vi "Measure vs B2Dv7.vi"() -> ()   [LabVIEW 2009]
doc: "This VI is an example operator panel.\n\nThe VI contains a table for the field values that may be configured manually, or loaded by checking the \"Prompt for File\" box. The data file should contain 3 columns of data, with each column delimited by a tab character.\n\nBefore the VI is executed, set the desired field units and coordinate system. Once the VI is started, follow the directions in the STATUS indicator to operate. Once a field value is achieved, it will be held indefinitely with no user intervention.\n\nThe present field is displayed in the selected units and coordinate system. The present field is queried once per second.\n\nIf a field point is specified that is outside the limits for the magnet, the VI will abort execution."
uses:
  <vilib>/Utility/file.llb/Read From Spreadsheet File (DBL).vi
panel:
  out "appended array":dbl[](array[numeric])=[0.2032200002460388, 90.00281939668669, 0.0, 0.0, 0.0, 0.0, 0.0, 0.0, 0.0, 0.0, -5.519596, 3403272764.31614]
  in  "Nr. of Accumulations":i32=5
  in  "X Axis":enum16{"B", "phi"}(ring)
  in  "Y Axis":T1(ring)=enum."HP (V)"
  out "XY Graph":T2(graph)={"measured data"=[0.10347000048323185, 0.19641000025456953, 0.29707, 0.396860000125989, 0.49694000010061584, 0.5974600000836876, 0.69603, 0.7960300000628118, 0.8974500000557136, 0.9966200002006783, 1.0970900000000001, 1.19673, 1.29725, 1.39698, 1.49648, 1.5970800000313075, 1.6969500000000002, 1.796500000027832, 1.8966700000263619, 1.9970400000000001, 2.0967400000238468, 2.196980000022758, 2.2964100000870924, 2.396280000020866, 2.49752000002002, 2.5961200000000004, 2.6964400000185433, 2.79707, 2.8966900000172613, 2.996840000016684, 3.0965000000000003, 3.1975700000000002, 3.29701, 3.39604, 3.496610000014299, 3.5968600000139013, 3.6964300000000003, 3.79707, 3.896600000012832, 3.99675000001251, 4.09672, 4.197190000011912, 4.29626, 4.3964799999999995, 4.496670000000001, 4.597080000010876, 4.696600000010646, 4.796870000010423, 4.896420000010211, 4.996820000010007, 4.903020000000001, 4.802990000010411, 4.703300000010631, 4.602810000043452, 4.50282, 4.403030000011356, 4.303300000011619, 4.203860000000001, 4.103380000012185, 4.002780000012492, 3.90318, 3.80358, 3.7033500000135007, 3.603490000013876, 3.5029500000142733, 3.40296, 3.3031700000605486, 3.2035800000156076, 3.10286, 3.0031200000665974, 2.90348, 2.8030600000000003, 2.7033300000000002, 2.603300000019207, 2.5035000000000003, 2.403530000020803, 2.3033300000000003, 2.2031300000000003, 2.1029400000237763, 2.003560000024956, 1.9032600000262705, 1.8035800000277225, 1.7029600000293605, 1.6035700000311803, 1.5032900000332605, 1.4031900000356332, 1.3032700000383652, 1.20313, 1.10329, 1.00339, 0.90345, 0.8029400000622712, 0.7036, 0.60275, 0.50339, 0.40294, 0.302990000165022, 0.2032200002460388], "measured data"=[-1.563466, -1.08216, -0.70321, -0.409586, -0.269864, -0.025948, 0.180408, 0.261814, 0.30081199999999997, -0.068092, -0.57451, -1.0081479999999998, -2.017134, -2.885122, -3.9488559999999997, -5.384270000000001, -7.012888, -8.998236, -11.360275999999999, -14.308696, -17.92829, -22.338188000000002, -28.965936000000003, -36.3468, -44.4973, -53.671188, -60.597266, -67.282196, -73.833424, -80.22503, -86.434398, -92.21979400000001, -97.86212, -103.22911199999999, -108.601316, -113.677622, -118.671314, -123.51419200000001, -128.272526, -132.90004199999998, -137.67711400000002, -142.21992799999998, -146.755386, -151.024336, -155.5273, -159.64799399999998, -163.87723999999997, -168.28429, -172.573372, -176.459164, -165.88622399999997, -156.948784, -147.825416, -141.431096, -136.35452, -131.8822, -127.589888, -123.29114200000001, -119.12121399999998, -115.08163, -111.252546, -107.22219799999999, -103.221754, -99.245906, -95.414286, -91.35763800000001, -87.32137, -83.26736600000001, -79.067984, -75.06495600000001, -70.80681200000001, -66.649182, -62.36449400000001, -58.344514000000004, -53.993213999999995, -50.057770000000005, -45.802158000000006, -42.018744, -38.010557999999996, -34.145004, -30.535152, -27.03073, -23.526186000000003, -20.238034, -17.346718, -14.648320000000002, -12.144, -9.910048, -7.987274, -6.390732, -5.077078, -4.234354, -3.7365180000000002, -3.579744, -3.8743040000000004, -4.396356, -5.0064459999999995, -5.519596]}
  in  "GPIB HP 2":string="13"
  in  "Wait between \nVectors":bool=TRUE
  in  "FieldRange":dbl=1.0
  in  "Change\nPID\n(DetermineSIMPID.vi)":bool
  in  "Wait between \nVectors (ms)":u32=4000
  out "measured data":dbl[][](array[numeric])=[[0.10347000048323185, 90.00553742914224, 0.0, 0.0, 0.0, 0.0, 0.0, 0.0, 0.0, 0.0, -1.563466, 3403269629.8467245], [0.19641000025456953, 89.99708284815114, 0.0, 0.0, 0.0, 0.0, 0.0, 0.0, 0.0, 0.0, -1.08216, 3403269661.616901], [0.29707, 90.0, 0.0, 0.0, 0.0, 0.0, 0.0, 0.0, 0.0, 0.0, -0.70321, 3403269694.1531544], [0.396860000125989, 90.00144372775037, 0.0, 0.0, 0.0, 0.0, 0.0, 0.0, 0.0, 0.0, -0.409586, 3403269726.399379], [0.49694000010061584, 89.99884702822263, 0.0, 0.0, 0.0, 0.0, 0.0, 0.0, 0.0, 0.0, -0.269864, 3403269759.355674], [0.5974600000836876, 90.00095898938018, 0.0, 0.0, 0.0, 0.0, 0.0, 0.0, 0.0, 0.0, -0.025948, 3403269791.685907], [0.69603, 90.0, 0.0, 0.0, 0.0, 0.0, 0.0, 0.0, 0.0, 0.0, 0.180408, 3403269823.3570733], [0.7960300000628118, 89.99928023090197, 0.0, 0.0, 0.0, 0.0, 0.0, 0.0, 0.0, 0.0, 0.261814, 3403269855.5922966], [0.8974500000557136, 90.00063842865353, 0.0, 0.0, 0.0, 0.0, 0.0, 0.0, 0.0, 0.0, 0.30081199999999997, 3403269888.02954], [0.9966200002006783, 90.0011498019206, 0.0, 0.0, 0.0, 0.0, 0.0, 0.0, 0.0, 0.0, -0.068092, 3403269919.970734], [1.0970900000000001, 90.0, 0.0, 0.0, 0.0, 0.0, 0.0, 0.0, 0.0, 0.0, -0.57451, 3403269952.1809545], [1.19673, 90.0, 0.0, 0.0, 0.0, 0.0, 0.0, 0.0, 0.0, 0.0, -1.0081479999999998, 3403269983.93713], [1.29725, 90.0, 0.0, 0.0, 0.0, 0.0, 0.0, 0.0, 0.0, 0.0, -2.017134, 3403270016.8654222], [1.39698, 90.0, 0.0, 0.0, 0.0, 0.0, 0.0, 0.0, 0.0, 0.0, -2.885122, 3403270049.372673], [1.49648, 90.0, 0.0, 0.0, 0.0, 0.0, 0.0, 0.0, 0.0, 0.0, -3.9488559999999997, 3403270081.84692], [1.5970800000313075, 89.9996412466532, 0.0, 0.0, 0.0, 0.0, 0.0, 0.0, 0.0, 0.0, -5.384270000000001, 3403270114.493184], [1.6969500000000002, 90.0, 0.0, 0.0, 0.0, 0.0, 0.0, 0.0, 0.0, 0.0, -7.012888, 3403270146.7094054], [1.796500000027832, 89.9996810699721, 0.0, 0.0, 0.0, 0.0, 0.0, 0.0, 0.0, 0.0, -8.998236, 3403270178.7226067], [1.8966700000263619, 90.00030208618006, 0.0, 0.0, 0.0, 0.0, 0.0, 0.0, 0.0, 0.0, -11.360275999999999, 3403270210.912825], [1.9970400000000001, 90.0, 0.0, 0.0, 0.0, 0.0, 0.0, 0.0, 0.0, 0.0, -14.308696, 3403270243.424076], [2.0967400000238468, 90.00027326125087, 0.0, 0.0, 0.0, 0.0, 0.0, 0.0, 0.0, 0.0, -17.92829, 3403270275.8403172], [2.196980000022758, 89.99973920664041, 0.0, 0.0, 0.0, 0.0, 0.0, 0.0, 0.0, 0.0, -22.338188000000002, 3403270308.229556], [2.2964100000870924, 89.99950099695167, 0.0, 0.0, 0.0, 0.0, 0.0, 0.0, 0.0, 0.0, -28.965936000000003, 3403270340.8998227], [2.396280000020866, 90.00023910302433, 0.0, 0.0, 0.0, 0.0, 0.0, 0.0, 0.0, 0.0, -36.3468, 3403270373.3240647], [2.49752000002002, 90.00022941069346, 0.0, 0.0, 0.0, 0.0, 0.0, 0.0, 0.0, 0.0, -44.4973, 3403270405.667299], [2.5961200000000004, 90.0, 0.0, 0.0, 0.0, 0.0, 0.0, 0.0, 0.0, 0.0, -53.671188, 3403270437.5914907], [2.6964400000185433, 90.00021248675851, 0.0, 0.0, 0.0, 0.0, 0.0, 0.0, 0.0, 0.0, -60.597266, 3403270469.938725], [2.79707, 90.0, 0.0, 0.0, 0.0, 0.0, 0.0, 0.0, 0.0, 0.0, -67.282196, 3403270502.9180226], [2.8966900000172613, 89.99980220258463, 0.0, 0.0, 0.0, 0.0, 0.0, 0.0, 0.0, 0.0, -73.833424, 3403270534.6661973], [2.996840000016684, 90.00019118731568, 0.0, 0.0, 0.0, 0.0, 0.0, 0.0, 0.0, 0.0, -80.22503, 3403270567.0204325], [3.0965000000000003, 90.0, 0.0, 0.0, 0.0, 0.0, 0.0, 0.0, 0.0, 0.0, -86.434398, 3403270599.029633], [3.1975700000000002, 90.0, 0.0, 0.0, 0.0, 0.0, 0.0, 0.0, 0.0, 0.0, -92.21979400000001, 3403270631.613891], [3.29701, 90.0, 0.0, 0.0, 0.0, 0.0, 0.0, 0.0, 0.0, 0.0, -97.86212, 3403270663.7301025], [3.39604, 90.0, 0.0, 0.0, 0.0, 0.0, 0.0, 0.0, 0.0, 0.0, -103.22911199999999, 3403270695.7623053], [3.496610000014299, 89.9998361390618, 0.0, 0.0, 0.0, 0.0, 0.0, 0.0, 0.0, 0.0, -108.601316, 3403270727.8155103], [3.5968600000139013, 89.99984070611725, 0.0, 0.0, 0.0, 0.0, 0.0, 0.0, 0.0, 0.0, -113.677622, 3403270760.053734], [3.6964300000000003, 90.0, 0.0, 0.0, 0.0, 0.0, 0.0, 0.0, 0.0, 0.0, -118.671314, 3403270792.41597], [3.79707, 90.0, 0.0, 0.0, 0.0, 0.0, 0.0, 0.0, 0.0, 0.0, -123.51419200000001, 3403270824.9382215], [3.896600000012832, 89.99985295955574, 0.0, 0.0, 0.0, 0.0, 0.0, 0.0, 0.0, 0.0, -128.272526, 3403270857.4414716], [3.99675000001251, 90.00014335592547, 0.0, 0.0, 0.0, 0.0, 0.0, 0.0, 0.0, 0.0, -132.90004199999998, 3403270889.768704], [4.09672, 90.0, 0.0, 0.0, 0.0, 0.0, 0.0, 0.0, 0.0, 0.0, -137.67711400000002, 3403270922.309958], [4.197190000011912, 89.99986349014576, 0.0, 0.0, 0.0, 0.0, 0.0, 0.0, 0.0, 0.0, -142.21992799999998, 3403270954.8822145], [4.29626, 90.0, 0.0, 0.0, 0.0, 0.0, 0.0, 0.0, 0.0, 0.0, -146.755386, 3403270987.409467], [4.3964799999999995, 90.0, 0.0, 0.0, 0.0, 0.0, 0.0, 0.0, 0.0, 0.0, -151.024336, 3403271020.102736], [4.496670000000001, 90.0, 0.0, 0.0, 0.0, 0.0, 0.0, 0.0, 0.0, 0.0, -155.5273, 3403271052.174943], [4.597080000010876, 90.00012463515866, 0.0, 0.0, 0.0, 0.0, 0.0, 0.0, 0.0, 0.0, -159.64799399999998, 3403271084.9372187], [4.696600000010646, 89.99987800583504, 0.0, 0.0, 0.0, 0.0, 0.0, 0.0, 0.0, 0.0, -163.87723999999997, 3403271116.9074154], [4.796870000010423, 89.99988055590518, 0.0, 0.0, 0.0, 0.0, 0.0, 0.0, 0.0, 0.0, -168.28429, 3403271149.044629], [4.896420000010211, 89.99988298434465, 0.0, 0.0, 0.0, 0.0, 0.0, 0.0, 0.0, 0.0, -172.573372, 3403271180.869811], [4.996820000010007, 90.00011466448564, 0.0, 0.0, 0.0, 0.0, 0.0, 0.0, 0.0, 0.0, -176.459164, 3403271213.3300567], [4.903020000000001, 90.0, 0.0, 0.0, 0.0, 0.0, 0.0, 0.0, 0.0, 0.0, -165.88622399999997, 3403271245.606284], [4.802990000010411, 90.00011929189841, 0.0, 0.0, 0.0, 0.0, 0.0, 0.0, 0.0, 0.0, -156.948784, 3403271277.7614994], [4.703300000010631, 90.0001218203804, 0.0, 0.0, 0.0, 0.0, 0.0, 0.0, 0.0, 0.0, -147.825416, 3403271310.397763], [4.602810000043452, 90.00024896000275, 0.0, 0.0, 0.0, 0.0, 0.0, 0.0, 0.0, 0.0, -141.431096, 3403271342.6319857], [4.50282, 90.0, 0.0, 0.0, 0.0, 0.0, 0.0, 0.0, 0.0, 0.0, -136.35452, 3403271374.9822206], [4.403030000011356, 89.99986987193022, 0.0, 0.0, 0.0, 0.0, 0.0, 0.0, 0.0, 0.0, -131.8822, 3403271407.48147], [4.303300000011619, 89.99986685618128, 0.0, 0.0, 0.0, 0.0, 0.0, 0.0, 0.0, 0.0, -127.589888, 3403271439.4496665], [4.203860000000001, 90.0, 0.0, 0.0, 0.0, 0.0, 0.0, 0.0, 0.0, 0.0, -123.29114200000001, 3403271471.840905], [4.103380000012185, 89.9998603693065, 0.0, 0.0, 0.0, 0.0, 0.0, 0.0, 0.0, 0.0, -119.12121399999998, 3403271503.7760987], [4.002780000012492, 89.9998568600335, 0.0, 0.0, 0.0, 0.0, 0.0, 0.0, 0.0, 0.0, -115.08163, 3403271536.004321], [3.90318, 90.0, 0.0, 0.0, 0.0, 0.0, 0.0, 0.0, 0.0, 0.0, -111.252546, 3403271568.6915894], [3.80358, 90.0, 0.0, 0.0, 0.0, 0.0, 0.0, 0.0, 0.0, 0.0, -107.22219799999999, 3403271600.5907793], [3.7033500000135007, 89.99984528662019, 0.0, 0.0, 0.0, 0.0, 0.0, 0.0, 0.0, 0.0, -103.221754, 3403271633.2210417], [3.603490000013876, 90.00015900080065, 0.0, 0.0, 0.0, 0.0, 0.0, 0.0, 0.0, 0.0, -99.245906, 3403271665.3602552], [3.5029500000142733, 90.00016356436579, 0.0, 0.0, 0.0, 0.0, 0.0, 0.0, 0.0, 0.0, -95.414286, 3403271697.578477], [3.40296, 90.0, 0.0, 0.0, 0.0, 0.0, 0.0, 0.0, 0.0, 0.0, -91.35763800000001, 3403271730.0967283], [3.3031700000605486, 89.99965308609904, 0.0, 0.0, 0.0, 0.0, 0.0, 0.0, 0.0, 0.0, -87.32137, 3403271762.6699853], [3.2035800000156076, 90.0001788492234, 0.0, 0.0, 0.0, 0.0, 0.0, 0.0, 0.0, 0.0, -83.26736600000001, 3403271795.0122194], [3.10286, 90.0, 0.0, 0.0, 0.0, 0.0, 0.0, 0.0, 0.0, 0.0, -79.067984, 3403271827.0044184], [3.0031200000665974, 89.99961842497461, 0.0, 0.0, 0.0, 0.0, 0.0, 0.0, 0.0, 0.0, -75.06495600000001, 3403271859.015619], [2.90348, 90.0, 0.0, 0.0, 0.0, 0.0, 0.0, 0.0, 0.0, 0.0, -70.80681200000001, 3403271891.048822], [2.8030600000000003, 90.0, 0.0, 0.0, 0.0, 0.0, 0.0, 0.0, 0.0, 0.0, -66.649182, 3403271923.7490916], [2.7033300000000002, 90.0, 0.0, 0.0, 0.0, 0.0, 0.0, 0.0, 0.0, 0.0, -62.36449400000001, 3403271956.3823547], [2.603300000019207, 89.99977991096104, 0.0, 0.0, 0.0, 0.0, 0.0, 0.0, 0.0, 0.0, -58.344514000000004, 3403271988.469563], [2.5035000000000003, 90.0, 0.0, 0.0, 0.0, 0.0, 0.0, 0.0, 0.0, 0.0, -53.993213999999995, 3403272020.721788], [2.403530000020803, 90.00023838179474, 0.0, 0.0, 0.0, 0.0, 0.0, 0.0, 0.0, 0.0, -50.057770000000005, 3403272052.866002], [2.3033300000000003, 90.0, 0.0, 0.0, 0.0, 0.0, 0.0, 0.0, 0.0, 0.0, -45.802158000000006, 3403272085.619277], [2.2031300000000003, 90.0, 0.0, 0.0, 0.0, 0.0, 0.0, 0.0, 0.0, 0.0, -42.018744, 3403272118.202535], [2.1029400000237763, 90.00027245560746, 0.0, 0.0, 0.0, 0.0, 0.0, 0.0, 0.0, 0.0, -38.010557999999996, 3403272150.6097755], [2.003560000024956, 90.0002859698712, 0.0, 0.0, 0.0, 0.0, 0.0, 0.0, 0.0, 0.0, -34.145004, 3403272183.1900334], [1.9032600000262705, 89.99969895978735, 0.0, 0.0, 0.0, 0.0, 0.0, 0.0, 0.0, 0.0, -30.535152, 3403272215.6872826], [1.8035800000277225, 90.00031767805983, 0.0, 0.0, 0.0, 0.0, 0.0, 0.0, 0.0, 0.0, -27.03073, 3403272247.8164954], [1.7029600000293605, 89.99966355181853, 0.0, 0.0, 0.0, 0.0, 0.0, 0.0, 0.0, 0.0, -23.526186000000003, 3403272279.875701], [1.6035700000311803, 90.00035730139322, 0.0, 0.0, 0.0, 0.0, 0.0, 0.0, 0.0, 0.0, -20.238034, 3403272312.562969], [1.5032900000332605, 90.00038113590533, 0.0, 0.0, 0.0, 0.0, 0.0, 0.0, 0.0, 0.0, -17.346718, 3403272344.8691993], [1.4031900000356332, 89.99959167483013, 0.0, 0.0, 0.0, 0.0, 0.0, 0.0, 0.0, 0.0, -14.648320000000002, 3403272377.095422], [1.3032700000383652, 90.00043963092462, 0.0, 0.0, 0.0, 0.0, 0.0, 0.0, 0.0, 0.0, -12.144, 3403272409.408653], [1.20313, 90.0, 0.0, 0.0, 0.0, 0.0, 0.0, 0.0, 0.0, 0.0, -9.910048, 3403272441.6508765], [1.10329, 90.0, 0.0, 0.0, 0.0, 0.0, 0.0, 0.0, 0.0, 0.0, -7.987274, 3403272473.618073], [1.00339, 90.0, 0.0, 0.0, 0.0, 0.0, 0.0, 0.0, 0.0, 0.0, -6.390732, 3403272506.1273236], [0.90345, 90.0, 0.0, 0.0, 0.0, 0.0, 0.0, 0.0, 0.0, 0.0, -5.077078, 3403272538.3895497], [0.8029400000622712, 89.99928642514372, 0.0, 0.0, 0.0, 0.0, 0.0, 0.0, 0.0, 0.0, -4.234354, 3403272570.79679], [0.7036, 90.0, 0.0, 0.0, 0.0, 0.0, 0.0, 0.0, 0.0, 0.0, -3.7365180000000002, 3403272602.6849785], [0.60275, 90.0, 0.0, 0.0, 0.0, 0.0, 0.0, 0.0, 0.0, 0.0, -3.579744, 3403272634.934203], [0.50339, 90.0, 0.0, 0.0, 0.0, 0.0, 0.0, 0.0, 0.0, 0.0, -3.8743040000000004, 3403272667.4324527], [0.40294, 90.0, 0.0, 0.0, 0.0, 0.0, 0.0, 0.0, 0.0, 0.0, -4.396356, 3403272699.4946585], [0.302990000165022, 89.99810898777213, 0.0, 0.0, 0.0, 0.0, 0.0, 0.0, 0.0, 0.0, -5.0064459999999995, 3403272731.8768964], [0.2032200002460388, 90.00281939668669, 0.0, 0.0, 0.0, 0.0, 0.0, 0.0, 0.0, 0.0, -5.519596, 3403272764.31614]]
  in  "Notes:":string="Datum: 31.10.11, Uhrzeit: 15:35, T0.3K,PID LOOPP 0.2, I  200: , Filter auf 12dB und 30Hz, PID Dämpfung:  P=0.6, D=6.2E-5, Laser 25°, 20mA, AOM 10mA, Sweep 0.15T/min,Winkelsweep 0.4° Winkelschritte, warten bei jedem Feldpunkt (measurevsB2Dv7.vi))4s, vectorsm3.txt,Kryo auf dem Boden, nach dem Ausbau des Systems, großer Abstand zwischen Faser und Cantilever(3V Signalamplitude)" caption="Notizen:"
  out "Messfile Refnum":refnum<file>
  in  "Measurement File":path=path "D:/UserData/Matthias/Messungen/STO_LAOR103/111104/111104_R103_90deg_M3.txt"
  in  "Sample name:":string="R103"
  in  "HP 1":bool=TRUE
  in  "GPIB HP":string="14"
  in  "HP 2":bool
  in  "LI 3":bool
  in  "GPIB L 3":string="8"
  in  "LI 2":bool
  in  "GPIB L 2":string="8"
  in  "LI 1":bool
  in  "GPIB L 1":string="8"
  out "Number of lines":i32=99
  in  "Operation":u16(ring)=1 items=["Stepwise", "Continous"]
  out "Ramp Rate along Vector (T/min)":dbl=0.24999999999999994 format="%.3f"
  out "Current Ramp Rate Z (T/min)":dbl=0.24999999874949982 format="%.3f"
  out "Current Ramp Rate Y (T/min)":dbl=2.500500087514032e-05 format="%.3f"
  in  "User defined Ramp Rate (T/min)":bool=TRUE
  in  "User defined Ramp Rate (T/min)":dbl=0.25 format="%.3f"
  in  "Z-Axis Communications Config":T3={"GPIB address"=22, "GPIB bus"=1, "connection ID"=refnum, "IP"="111.111.111.1", "Active Comm Interface"=0, "Serial Port"="", "Programmer Type"=0} {"Programmer Type" items=["Model 430", "Model 420"]; "Active Comm Interface" items=["TCP/IP (Model 430 Only)", "RS232", "IEEE488"]}
  in  "Max Ramp Rate - Y Axis (A/s)":dbl=0.055 format="%.3f"
  in  "Max Ramp Rate - Z Axis (A/s)":dbl=0.19 format="%.3f"
  in  "Magnitude Limit (kG)":dbl=45.1 format="%.3f"
  in  "Y-Axis Communications Config":T3={"GPIB address"=22, "GPIB bus"=1, "connection ID"=refnum, "IP"="111.111.111.2", "Active Comm Interface"=0, "Serial Port"="", "Programmer Type"=0} {"Programmer Type" items=["Model 430", "Model 420"]; "Active Comm Interface" items=["TCP/IP (Model 430 Only)", "RS232", "IEEE488"]}
  out "Cartesian Display (T)":T4={"Y-Axis Field (T)"=0.01746, "Z-Axis Field (T)"=0.99986} {"Z-Axis Field (T)" format="%.3f"; "Y-Axis Field (T)" format="%.3f"}
  in  "Starting index":i32=99
  in  "Normal color":u32(colorbox)=11711154
  in  "Highlight color":u32(colorbox)=16711680
  in  "Prompt for File?":bool=TRUE
  out "Continue Execution?":bool=TRUE
  out "error out":T5
  in  "error in":T5
  out "STATUS":string="Zeroing vector."
  in  "Ramping Control":u16(ring)=4 items=["NEXT VECTOR", "RAMPING", "HOLDING", "PAUSE", "ZERO"]
  out "Cartesian Display (kG)":T6 {"Z-Axis Field (kG)" format="%.3f"; "Y-Axis Field (kG)" format="%.3f"}
  in  "Field Values":string[][](table)=[["0.1000", "90.0000"], ["0.2000", "90.0000"], ["0.3000", "90.0000"], ["0.4000", "90.0000"], ["0.5000", "90.0000"], ["0.6000", "90.0000"], ["0.7000", "90.0000"], ["0.8000", "90.0000"], ["0.9000", "90.0000"], ["1.0000", "90.0000"], ["1.1000", "90.0000"], ["1.2000", "90.0000"], ["1.3000", "90.0000"], ["1.4000", "90.0000"], ["1.5000", "90.0000"], ["1.6000", "90.0000"], ["1.7000", "90.0000"], ["1.8000", "90.0000"], ["1.9000", "90.0000"], ["2.0000", "90.0000"], ["2.1000", "90.0000"], ["2.2000", "90.0000"], ["2.3000", "90.0000"], ["2.4000", "90.0000"], ["2.5000", "90.0000"], ["2.6000", "90.0000"], ["2.7000", "90.0000"], ["2.8000", "90.0000"], ["2.9000", "90.0000"], ["3.0000", "90.0000"], ["3.1000", "90.0000"], ["3.2000", "90.0000"], ["3.3000", "90.0000"], ["3.4000", "90.0000"], ["3.5000", "90.0000"], ["3.6000", "90.0000"], ["3.7000", "90.0000"], ["3.8000", "90.0000"], ["3.9000", "90.0000"], ["4.0000", "90.0000"], ["4.1000", "90.0000"], ["4.2000", "90.0000"], ["4.3000", "90.0000"], ["4.4000", "90.0000"], ["4.5000", "90.0000"], ["4.6000", "90.0000"], ["4.7000", "90.0000"], ["4.8000", "90.0000"], ["4.9000", "90.0000"], ["5.0000", "90.0000"], ["4.9000", "90.0000"], ["4.8000", "90.0000"], ["4.7000", "90.0000"], ["4.6000", "90.0000"], ["4.5000", "90.0000"], ["4.4000", "90.0000"], ["4.3000", "90.0000"], ["4.2000", "90.0000"], ["4.1000", "90.0000"], ["4.0000", "90.0000"], ["3.9000", "90.0000"], ["3.8000", "90.0000"], ["3.7000", "90.0000"], ["3.6000", "90.0000"], ["3.5000", "90.0000"], ["3.4000", "90.0000"], ["3.3000", "90.0000"], ["3.2000", "90.0000"], ["3.1000", "90.0000"], ["3.0000", "90.0000"], ["2.9000", "90.0000"], ["2.8000", "90.0000"], ["2.7000", "90.0000"], ["2.6000", "90.0000"], ["2.5000", "90.0000"], ["2.4000", "90.0000"], ["2.3000", "90.0000"], ["2.2000", "90.0000"], ["2.1000", "90.0000"], ["2.0000", "90.0000"], ["1.9000", "90.0000"], ["1.8000", "90.0000"], ["1.7000", "90.0000"], ["1.6000", "90.0000"], ["1.5000", "90.0000"], ["1.4000", "90.0000"], ["1.3000", "90.0000"], ["1.2000", "90.0000"], ["1.1000", "90.0000"], ["1.0000", "90.0000"], ["0.9000", "90.0000"], ["0.8000", "90.0000"], ["0.7000", "90.0000"], ["0.6000", "90.0000"], ["0.5000", "90.0000"], ["0.4000", "90.0000"], ["0.3000", "90.0000"], ["0.2000", "90.0000"], ["0.1000", "90.0000"]]
  out "Switch Heaters":bool=TRUE
  out "Polar Display (T)":T7={"q (degrees)"=90.0, "Field Magnitude (T)"=0.00023} {"Field Magnitude (T)" format="%.3f"; "q (degrees)" format="%.3f"}
  out "Polar Display (kG)":T8 {"Field Magnitude (kG)" format="%.3f"; "q (degrees)" format="%.3f"}
  in  "Coordinate System":u16(ring)=1 items=["Cartesian", "Polar"]
  in  "Magnetic Field Units":u16(ring)=1 items=["kG", "Tesla"]
  # "Measurement Display"
  # "Measurement Settings"
  # "Magnet Settings"
  # "Max Ramp Rate z: 1.27 T/min\nMax Ramp Rate y: 0.17 T/min"
  # "Devices"
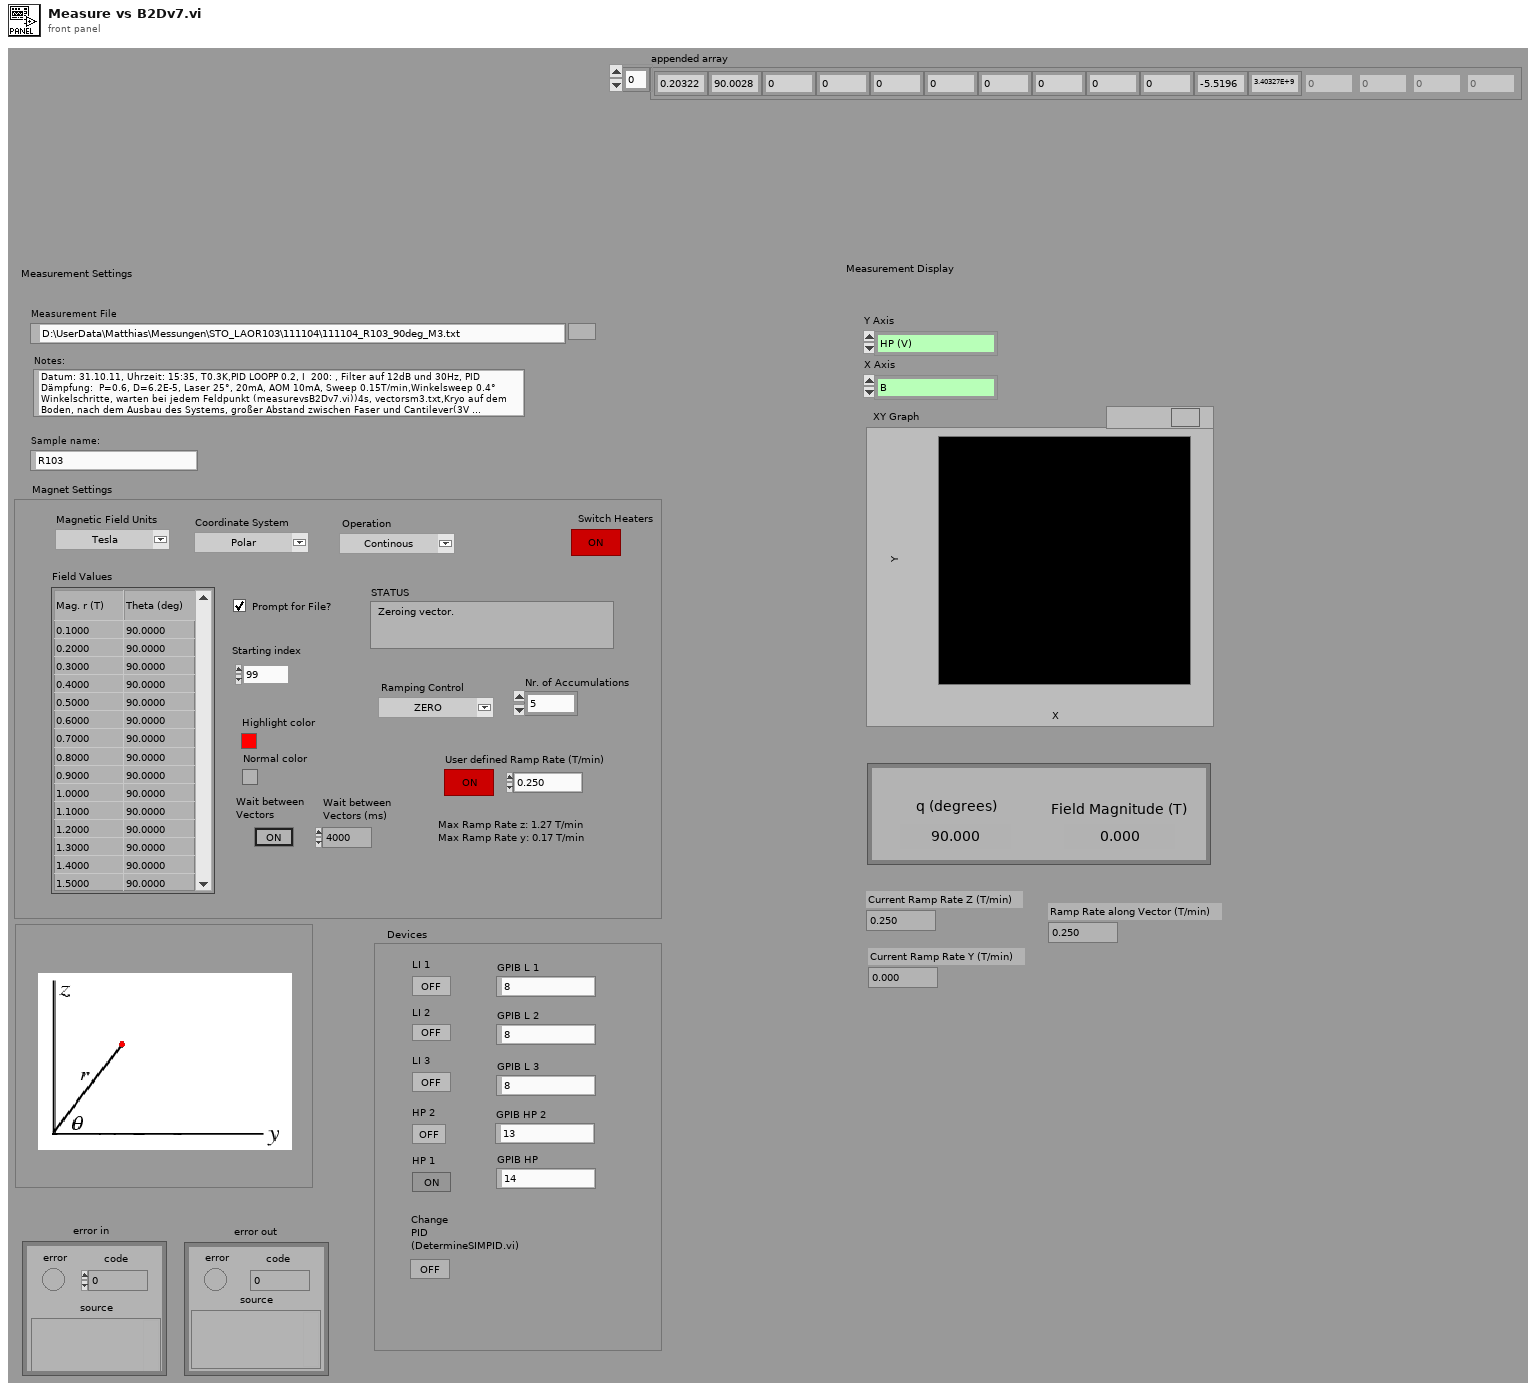
[diagram p1: front panel]
types:
  T1 = enum16{"B", "phi", "LI 1 Vx", "LI 1 phase", "LI 2 Vx", "LI 2 phase", "LI 3 Vx", "LI 3 phase", "LI 4 Vx", "LI 4 phase", "HP (V)"}
  T2 = cluster{"measured data":dbl[], "measured data":dbl[]}
  T3 = cluster{"GPIB address":i16, "GPIB bus":i16, "connection ID":refnum<k5>, "IP":string, "Active Comm Interface":u16, "Serial Port":refnum<visa-resource-name>, "Programmer Type":u16}
  T4 = cluster{"Y-Axis Field (T)":dbl, "Z-Axis Field (T)":dbl}
  T5 = cluster{"error":bool, "code":i32, "source":string}
  T6 = cluster{"Y-Axis Field (kG)":dbl, "Z-Axis Field (kG)":dbl}
  T7 = cluster{"q (degrees)":dbl, "Field Magnitude (T)":dbl}
  T8 = cluster{"q (degrees)":dbl, "Field Magnitude (kG)":dbl}
  T9 = enum16{"", "RAMPING", "HOLDING", "PAUSED", "MANUAL UP", "MANUAL DOWN", "ZEROING CURRENT", "QUENCH DETECTED", "HEATING SWITCH"}
  T10 = enum16{"", "RAMPING", "HOLDING", "PAUSED", "MANUAL UP", "MANUAL DOWN", "ZEROING CURRENT", "QUENCH DETECTED", "HEATING SWITCH", "AT ZER0", "COOLING SWITCH"}
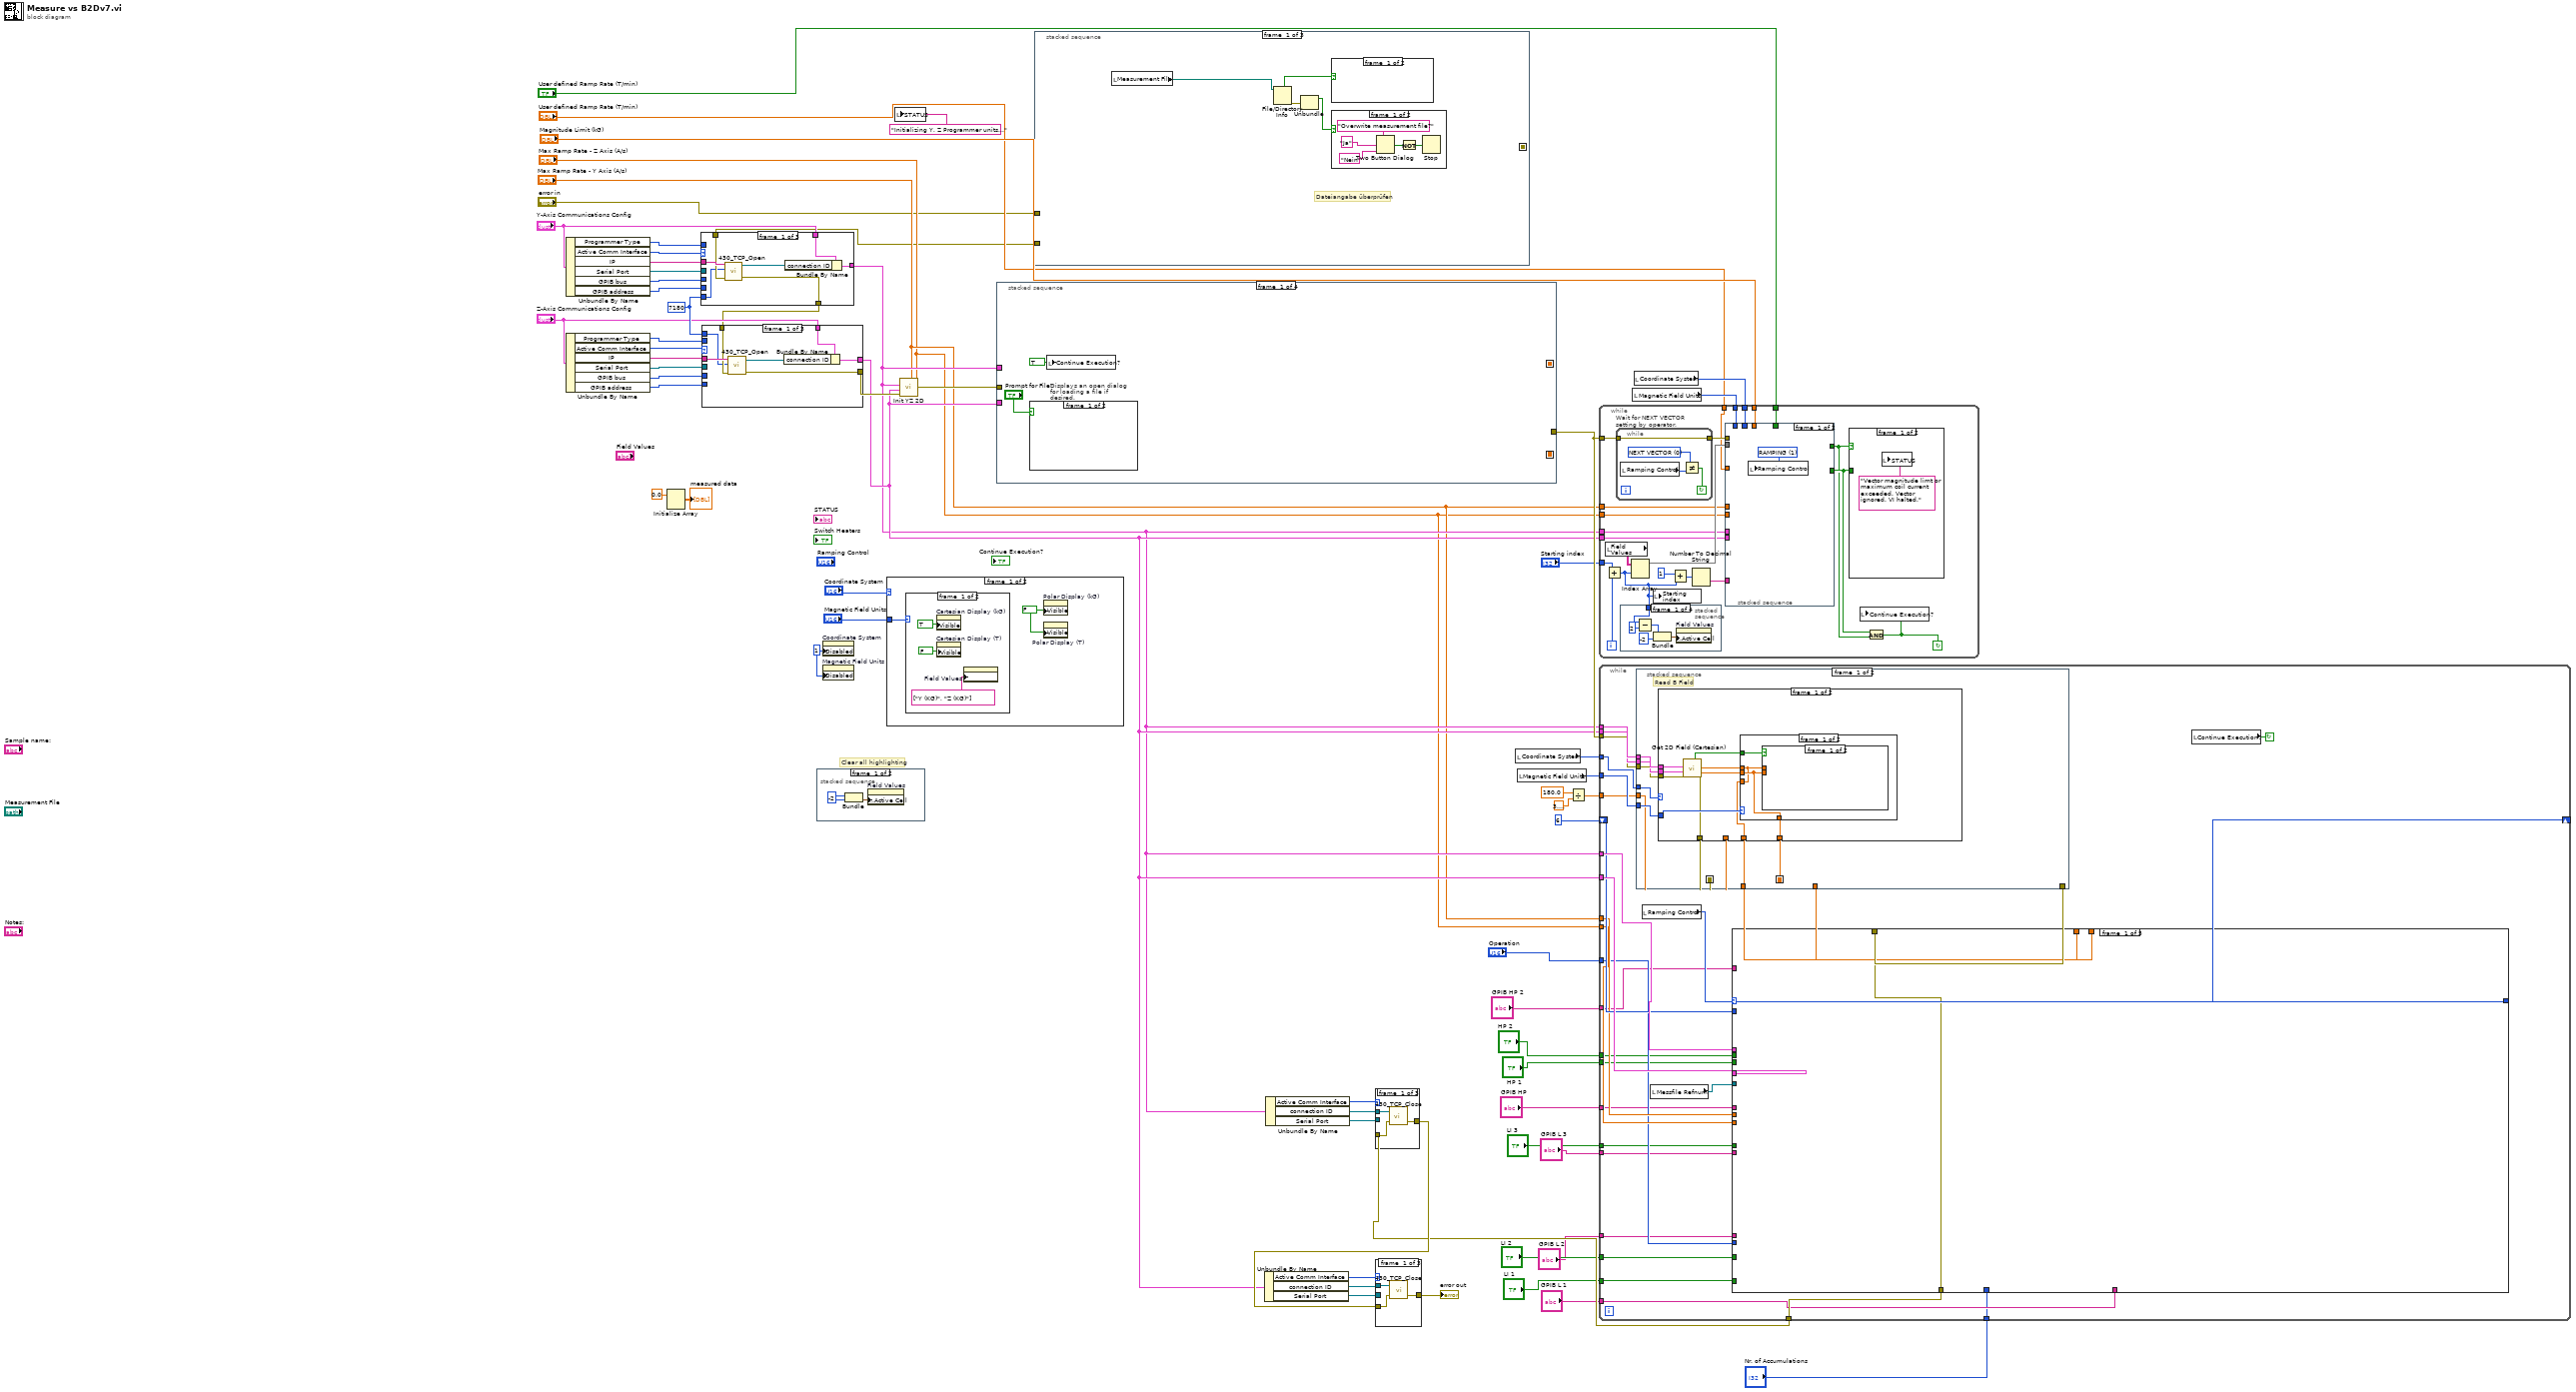
[diagram p0: block diagram]
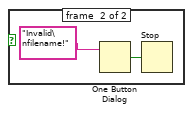
[diagram p3: hidden frame]
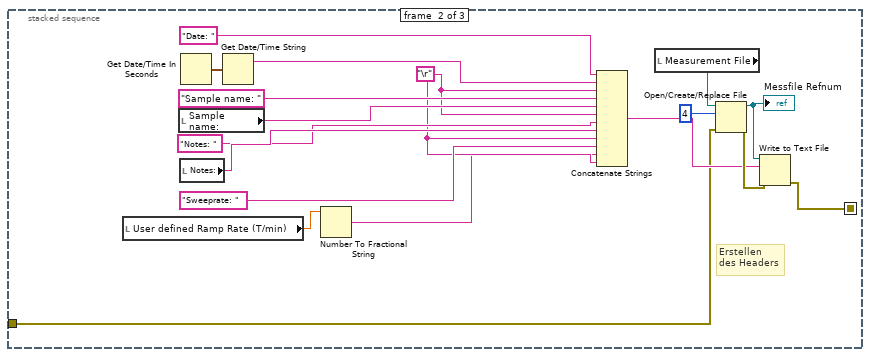
[diagram p4: hidden frame]
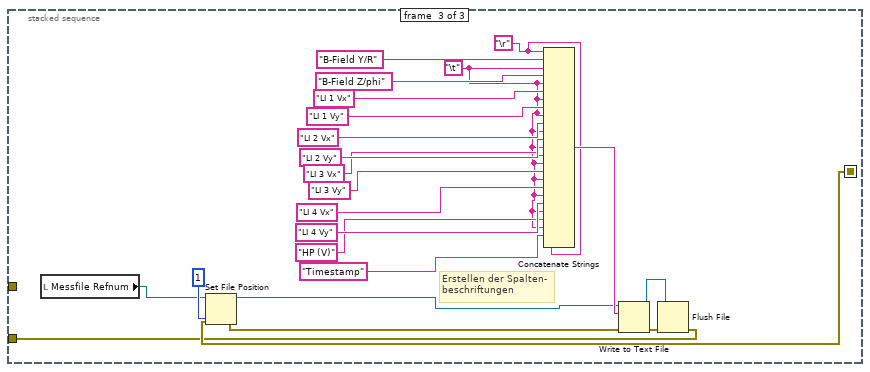
[diagram p5: hidden frame]
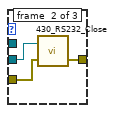
[diagram p6: hidden frame]
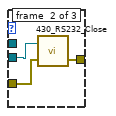
[diagram p8: hidden frame]
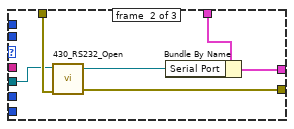
[diagram p10: hidden frame]
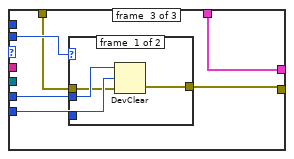
[diagram p11: hidden frame]
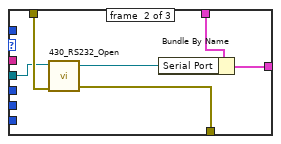
[diagram p13: hidden frame]
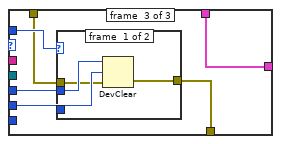
[diagram p14: hidden frame]
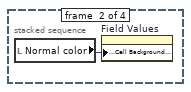
[diagram p16: hidden frame]
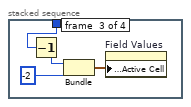
[diagram p17: hidden frame]
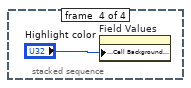
[diagram p18: hidden frame]
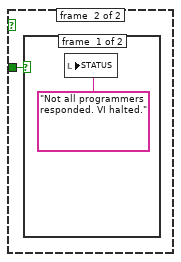
[diagram p19: hidden frame]
diagram:
  w49 = 7180 ("TCP Port")
  w62 = u8 1 ("Write Attribute")
  # "Clear all highlighting"
  n1 = Unbundle By Name("Z-Axis Communications Config") -> ("Programmer Type"=w25:u16, "Active Comm Interface"=w48:u16, "IP"=w45:string, "Serial Port"=w44:refnum<visa-resource-name>, "GPIB bus"=w24:i16, "GPIB address"=w23:i16)
  n2 = Unbundle By Name("Y-Axis Communications Config") -> ("Programmer Type"=w19:u16, "Active Comm Interface"=w47:u16, "IP"=w46:string, "Serial Port"=w43:refnum<visa-resource-name>, "GPIB bus"=w20:i16, "GPIB address"=w21:i16)
  n3 = Initialize Array(0.0 ("element")) -> (→"measured data":dbl[][])  [unwired: 2 in]
  n4 = stacked-sequence {
    frame #0 {
      w65 = -2
      n5 = Bundle(w65, w65) -> (w66:cluster{i32, i32})  [unwired: 1 in]
      n6 = property on="Field Values" class="Tbl (strict)"("Active Cell:Active Cell"=w66) -> ()  [unwired: 2 in, 2 out]
    }
    frame #1 {
      n7 = property on="Field Values" class="Tbl (strict)"("Active Cell:Cell Background Color"="Normal color") -> ()  [unwired: 2 in, 2 out]
    }
  }
  n8 = property on="Coordinate System" class="Ring (strict)"("Disabled"=w62) -> ()  [unwired: 2 in, 2 out]
  n9 = property on="Magnetic Field Units" class="Ring (strict)"("Disabled"=w62) -> ()  [unwired: 2 in, 2 out]
  n10 = case shown="0, Default" "Coordinate System" {
    tunnel: "Magnetic Field Units" -> [w69 w77]
    frame #0 {
      w68 = FALSE ("Write Attribute")
      (unwired) FALSE ("Write Attribute")
      (unwired) TRUE ("Write Attribute")
      n11 = case shown="1" w69 {
        frame #0 {
          n12 = property on="Cartesian Display (kG)" class="Cluster (strict)"("Visible"=TRUE ("Write Attribute")) -> ()  [unwired: 2 in, 2 out]
          n13 = property on="Cartesian Display (T)" class="Cluster (strict)"("Visible"=FALSE ("Write Attribute")) -> ()  [unwired: 2 in, 2 out]
          n14 = property on="Field Values" class="Tbl (strict)"("Column Header Strings[]"=string[] ["Y (KG)", "Z (KG)"] ("Write Attribute")) -> ()  [unwired: 2 in, 2 out]
        }
        frame #1 {
          n15 = property on="Cartesian Display (kG)" class="Cluster (strict)"("Visible"=FALSE ("Write Attribute")) -> ()  [unwired: 2 in, 2 out]
          n16 = property on="Cartesian Display (T)" class="Cluster (strict)"("Visible"=TRUE ("Write Attribute")) -> ()  [unwired: 2 in, 2 out]
          n17 = property on="Field Values" class="Tbl (strict)"("Column Header Strings[]"=string[] ["Y (T)", "Z (T)"] ("Write Attribute")) -> ()  [unwired: 2 in, 2 out]
        }
      }
      n18 = property on="Polar Display (kG)" class="Clust (strict)"("Visible"=w68) -> ()  [unwired: 2 in, 2 out]
      n19 = property on="Polar Display (T)" class="Clust (strict)"("Visible"=w68) -> ()  [unwired: 2 in, 2 out]
    }
    frame #1 {
      (unwired) FALSE ("Write Attribute")
      (unwired) TRUE ("Write Attribute")
      w76 = FALSE ("Write Attribute")
      n20 = case shown="1" w77 {
        frame #0 {
          n21 = property on="Polar Display (kG)" class="Clust (strict)"("Visible"=TRUE ("Write Attribute")) -> ()  [unwired: 2 in, 2 out]
          n22 = property on="Polar Display (T)" class="Clust (strict)"("Visible"=FALSE ("Write Attribute")) -> ()  [unwired: 2 in, 2 out]
          n23 = property on="Field Values" class="Tbl (strict)"("Column Header Strings[]"=string[] ["Mag. r (KG)", "Theta (deg)"] ("Write Attribute")) -> ()  [unwired: 2 in, 2 out]
        }
        frame #1 {
          n24 = property on="Polar Display (kG)" class="Clust (strict)"("Visible"=FALSE ("Write Attribute")) -> ()  [unwired: 2 in, 2 out]
          n25 = property on="Polar Display (T)" class="Clust (strict)"("Visible"=TRUE ("Write Attribute")) -> ()  [unwired: 2 in, 2 out]
          n26 = property on="Field Values" class="Tbl (strict)"("Column Header Strings[]"=string[] ["Mag. r (T)", "Theta (deg)"] ("Write Attribute")) -> ()  [unwired: 2 in, 2 out]
        }
      }
      n27 = property on="Cartesian Display (kG)" class="Cluster (strict)"("Visible"=w76) -> ()  [unwired: 2 in, 2 out]
      n28 = property on="Cartesian Display (T)" class="Cluster (strict)"("Visible"=w76) -> ()  [unwired: 2 in, 2 out]
    }
  }
  n29 = local write "STATUS"("Initializing Y, Z Programmer units..." ("STATUS")) -> ()
  n30 = stacked-sequence {
    seq-local: [_ w95 _] -> [_ _ w114]
    tunnel: "error in" -> [_ w96 _]
    tunnel: [_ _ w113] -> w14
    frame #0 {
      # "Dateiangabe überprüfen"
      n31 = local read "Measurement File"() -> (w87:path)
      n32 = File/Directory Info(path=w87) -> (directory=w85:bool, error out=w86:errorcluster)  [unwired: 1 in, 5 out]
      n33 = Unbundle(w86) -> ("status"=w84:bool)  [unwired: 2 out]
      n34 = case shown="False" w85 {
        frame #0 {
        }
        frame #1 {
          n35 = One Button Dialog(message="Invalid\nfilename!") -> (true=w93:bool)  [unwired: 1 in]
          n36 = Stop(stop? (T)=w93) -> ()
        }
      }
      n37 = case shown="False" w84 {
        frame #0 {
          n38 = Two Button Dialog(message="Overwrite measurement file?", 1:"Nein", 2:"Ja") -> (T button?=w89:bool)
          n39 = Not(x=w89) -> (.not. x?=w88:bool)
          n40 = Stop(stop? (T)=w88) -> ()
        }
        frame #1 {
        }
      }
    }
    frame #1 {
      w99 = "\r"
      # "Erstellen\ndes Headers"
      n41 = local read "User defined Ramp Rate (T/min)"() -> (w98:dbl)
      n42 = local read "Sample name:"() -> (w105:string)
      n43 = local read "Notes:"() -> (w107:string)
      n44 = Get Date/Time In Seconds() -> (seconds since 1Jan1904=w101:timestamp)
      n45 = Get Date/Time String(seconds (now)=w101) -> (date string=w103:string)  [unwired: 2 in, 1 out]
      n46 = Number To Fractional String(number=w98) -> (F-format string=w97:string)  [unwired: 3 in]
      n47 = Concatenate Strings("Date: ", w103, w99, "Sample name: ", w105, w99, "Notes: ", w107, w99, "Sweeprate: ", w97, w99) -> (w111:string)
      n48 = local read "Measurement File"() -> (w108:path)
      n49 = Open/Create/Replace File(file path (use dialog)=w108, error in=w96, operation (0:open)=4) -> (refnum out=w110:refnum<file>, error out=w112:errorcluster)  [unwired: 3 in, 1 out]
      "Messfile Refnum" <- w110
      n50 = Write to Text File(file (use dialog)=w110, text=w111, error in=w112) -> (error out=w95:errorcluster)  [unwired: 1 in, 2 out]
    }
    frame #2 {
      w117 = "\t"
      w115 = "\r"
      # "Erstellen der Spalten-\nbeschriftungen"
      n51 = local read "Messfile Refnum"() -> (w124:refnum<file>)
      n52 = Set File Position(refnum=w124, from (0:start)=1, error in=w114) -> (refnum out=w130:refnum<file>, error out=w132:errorcluster)  [unwired: 1 in]
      n53 = Concatenate Strings(w115, "B-Field Y/R", w117, "B-Field Z/phi", w117, "LI 1 Vx", w117, "LI 1 Vy", w117, "LI 2 Vx", w117, "LI 2 Vy", w117, "LI 3 Vx", w117, "LI 3 Vy", w117, "LI 4 Vx", w117, "LI 4 Vy", w117, "HP (V)", w117, "Timestamp", w115) -> (w131:string)
      n54 = Write to Text File(file (use dialog)=w130, text=w131, error in=w132) -> (refnum out=w134:refnum<file>, error out=w133:errorcluster)  [unwired: 1 in, 1 out]
      n55 = Flush File(refnum=w134, error in=w133) -> (error out=w113:errorcluster)  [unwired: 1 out]
    }
  }
  n56 = case shown="2" w47 {
    tunnel: w46 -> [w142 _ _]
    tunnel: w14 -> [w141 w148 w150]
    tunnel: "Y-Axis Communications Config" -> [w140 w143 w154]
    tunnel: [w138 w146 w154] -> w32
    tunnel: [w137 w147 w149] -> w22
    tunnel: w49 -> [w136 _ _]
    tunnel: w43 -> [_ w144 _]
    tunnel: w21 -> [_ _ w153]
    tunnel: w20 -> [_ _ w152]
    tunnel: w19 -> [_ _ w151]
    frame #0 {
      n57 = call <userlib>:"430_TCP_Open.vi"("IP Address"=w142, "TCP Port"=w136, "error in (no error)"=w141) -> ("connection ID"=w139:refnum<k5>, "error out"=w137:errorcluster)  [unwired: 3 in, 1 out]
      n58 = Bundle By Name(cluster=w140, "connection ID"=w139) -> (w138:T3)
    }
    frame #1 {
      n59 = call <userlib>:"430_RS232_Open.vi"("VISA resource name"=w144, "error in (no error)"=w148) -> ("VISA resource name out"=w145:refnum<visa-resource-name>, "error out"=w147:errorcluster)  [unwired: 5 in]
      n60 = Bundle By Name(cluster=w143, "Serial Port"=w145) -> (w146:T3)
    }
    frame #2 {
      n61 = case shown="0, Default" w151 {
        tunnel: w152 -> [w158 _]
        tunnel: w153 -> [w157 _]
        tunnel: w150 -> [w156 w159]
        tunnel: [w155 w159] -> w149
        frame #0 {
          n62 = DevClear(2:w156, 3:w157, 4:w158) -> (0:w155:errorcluster)  [unwired: 1 out]
        }
        frame #1 {
        }
      }
    }
  }
  n63 = case shown="2" w48 {
    tunnel: w45 -> [w166 _ _]
    tunnel: w22 -> [w165 w172 w174]
    tunnel: [w164 w171 w173] -> w42
    tunnel: "Z-Axis Communications Config" -> [w163 w169 w178]
    tunnel: [w161 w170 w178] -> w33
    tunnel: w49 -> [w160 _ _]
    tunnel: w44 -> [_ w167 _]
    tunnel: w25 -> [_ _ w177]
    tunnel: w24 -> [_ _ w176]
    tunnel: w23 -> [_ _ w175]
    frame #0 {
      n64 = call <userlib>:"430_TCP_Open.vi"("IP Address"=w166, "TCP Port"=w160, "error in (no error)"=w165) -> ("connection ID"=w162:refnum<k5>, "error out"=w164:errorcluster)  [unwired: 3 in, 1 out]
      n65 = Bundle By Name(cluster=w163, "connection ID"=w162) -> (w161:T3)
    }
    frame #1 {
      n66 = call <userlib>:"430_RS232_Open.vi"("VISA resource name"=w167, "error in (no error)"=w172) -> ("VISA resource name out"=w168:refnum<visa-resource-name>, "error out"=w171:errorcluster)  [unwired: 5 in]
      n67 = Bundle By Name(cluster=w169, "Serial Port"=w168) -> (w170:T3)
    }
    frame #2 {
      n68 = case shown="0, Default" w177 {
        tunnel: w176 -> [w182 _]
        tunnel: w175 -> [w181 _]
        tunnel: w174 -> [w180 w183]
        tunnel: [w179 w183] -> w173
        frame #0 {
          n69 = DevClear(2:w180, 3:w181, 4:w182) -> (0:w179:errorcluster)  [unwired: 1 out]
        }
        frame #1 {
        }
      }
    }
  }
  n70 = call <userlib>:"Init YZ 2D.vi"("Max Ramp Rate Z-axis"="Max Ramp Rate - Z Axis (A/s)", "Max Ramp Rate Y-axis"="Max Ramp Rate - Y Axis (A/s)", "error in"=w42, "Z-Axis Communications Config"=w33, "Y-Axis Communications Config"=w32) -> ("error out"=w60:T5)  [unwired: 5 in]
  n71 = stacked-sequence {
    seq-local: [_ w191 _ _] -> [_ _ w238 _]
    seq-local: [_ w190 _ _] -> [_ _ w237 _]
    tunnel: w33 -> [_ w193 _ _]
    tunnel: w60 -> [_ w194 _ _]
    tunnel: [_ w189 _ _] -> w56
    tunnel: w32 -> [_ w192 _ _]
    frame #0 {
      n72 = case "Displays an open dialog for loading a file if desired." shown="True" "Prompt for File?" {
        frame #0 {
        }
        frame #1 {
          n73 = call-poly <vilib>:"Read From Spreadsheet File.vi"() -> ("all rows"=w188:dbl[][])  [unwired: 7 in, 4 out]
          n74 = Number To Fractional String(number=w188, precision (6)=i16 4) -> (F-format string=w187:string[][])  [unwired: 2 in]
          n75 = local write "Field Values"(w187) -> ()
        }
      }
      n76 = local write "Continue Execution?"(TRUE ("Continue Execution?")) -> ()
    }
    frame #1 {
      w202 = u16 3 items=["NEXT VECTOR", "RAMPING", "HOLDING", "PAUSE", "ZERO"] ("Ramping Control")
      n77 = call <userlib>:"Get Switch Present.vi"("error in"=w194, "Communications Config"=w192) -> ("error out"=w198:T5, "Switch Present?"=w199:bool)
      n78 = case shown="True" w199 {
        tunnel: w198 -> [w220 w229]
        tunnel: w192 -> [_ w222]
        tunnel: [0.0 w226] -> w190
        tunnel: [w220 w228] -> w197
        frame #0 {
        }
        frame #1 {
          n79 = call <userlib>:"Get Switch Heater Time.vi"("error in"=w229, "Communications Config"=w222) -> ("error out"=w225:T5, "Switch Heating Time (secs)"=w227:dbl)
          n80 = call <userlib>:"Get Switch Heater.vi"("error in"=w225, "Communications Config"=w222) -> ("error out"=w224:T5, "Switch Heater Indicator"=w223:bool)
          n81 = case shown="False" w223 {
            tunnel: [w234 w235] -> w228
            tunnel: w227 -> [w232 _]
            tunnel: [w232 0.0] -> w226
            tunnel: w224 -> [w230 w235]
            tunnel: w222 -> [w231 _]
            frame #0 {
              n82 = call <userlib>:"Set Switch Heater.vi"("error in"=w230, "Switch Heater Control"=TRUE, "Communications Config"=w231) -> ("error out"=w234:T5)
            }
            frame #1 {
            }
          }
        }
      }
      n83 = call <userlib>:"Get Switch Present.vi"("error in"=w197, "Communications Config"=w193) -> ("error out"=w195:T5, "Switch Present?"=w196:bool)
      n84 = case shown="True" w196 {
        tunnel: w195 -> [w203 w212]
        tunnel: w193 -> [_ w205]
        tunnel: [0.0 w209] -> w191
        tunnel: [w203 w211] -> w189
        frame #0 {
        }
        frame #1 {
          n85 = call <userlib>:"Get Switch Heater Time.vi"("error in"=w212, "Communications Config"=w205) -> ("error out"=w208:T5, "Switch Heating Time (secs)"=w210:dbl)
          n86 = call <userlib>:"Get Switch Heater.vi"("error in"=w208, "Communications Config"=w205) -> ("error out"=w207:T5, "Switch Heater Indicator"=w206:bool)
          n87 = case shown="False" w206 {
            tunnel: [w213 w218] -> w211
            tunnel: w210 -> [w216 _]
            tunnel: [w216 0.0] -> w209
            tunnel: w207 -> [w214 w218]
            tunnel: w205 -> [w215 _]
            frame #0 {
              n88 = call <userlib>:"Set Switch Heater.vi"("error in"=w214, "Switch Heater Control"=TRUE, "Communications Config"=w215) -> ("error out"=w213:T5)
            }
            frame #1 {
            }
          }
        }
      }
      n89 = local write "Ramping Control"(w202) -> ()
      n90 = local write "Switch Heaters"(TRUE ("Switch Heater Control")) -> ()
      n91 = property on="Switch Heaters" class="Boolean (strict)"("Disabled"=u8 1 ("Write Attribute")) -> ()  [unwired: 2 in, 2 out]
    }
    frame #2 {
      n92 = Max & Min(x=w238, y=w237) -> (max(x,y)=w239:dbl)  [unwired: 1 out]
      n93 = local write "STATUS"("Heating switches..." ("STATUS")) -> ()
      n94 = Add(x=w239, y=2) -> (x+y=w243:dbl)
      n95 = property on="Ramping Control" class="Ring (strict)"("Disabled"=u8 1 ("Write Attribute")) -> ()  [unwired: 2 in, 2 out]
      n96 = Multiply(x=w243, y=1000) -> (x*y=w242:dbl)
      n97 = Wait (ms)(milliseconds to wait=w242) -> ()  [unwired: 1 out]
    }
    frame #3 {
      n98 = property on="Ramping Control" class="Ring (strict)"("Disabled"=u8 0 ("Write Attribute")) -> ()  [unwired: 2 in, 2 out]
      n99 = local write "STATUS"("Ready to ramp to first vector. Set Ramping Mode to NEXT VECTOR to begin." ("STATUS")) -> ()
      n100 = local read "Field Values"() -> (w248:string[][])
      n101 = Array Size(array=w248) -> (size(s)=w247:i32[])
      n102 = Index Array(array=w247, index=0) -> (element=→"Number of lines":i32)
    }
  }
  n103 = Unbundle By Name(w33) -> ("Active Comm Interface"=w39:u16, "connection ID"=w38:refnum<k5>, "Serial Port"=w37:refnum<visa-resource-name>)
  n104 = Unbundle By Name(w32) -> ("Active Comm Interface"=w40:u16, "connection ID"=w36:refnum<k5>, "Serial Port"=w35:refnum<visa-resource-name>)
  n105 = local read "Coordinate System"() -> (w57:u16)
  n106 = local read "Magnetic Field Units"() -> (w55:u16)
  n107 = Divide(x=180.0, y=3.141592653589793) -> (x/y=w52:dbl)
  n108 = while {
    shift-left: u16 6 ("Ramping Control") -> [w271]
    shift-right: [w272] -> _
    tunnel: [w274] -> w34
    tunnel: w33 -> [w275]
    tunnel: w32 -> [w276]
    tunnel: w52 -> [w278]
    tunnel: w55 -> [w279]
    tunnel: w56 -> [w280]
    tunnel: w33 -> [w281]
    tunnel: w32 -> [w282]
    tunnel: w57 -> [w266]
    tunnel: "Max Ramp Rate - Y Axis (A/s)" -> [w270]
    tunnel: "Max Ramp Rate - Z Axis (A/s)" -> [w269]
    tunnel: "Operation" -> [w268]
    tunnel: "LI 1" -> [w263]
    tunnel: "LI 2" -> [w262]
    tunnel: "LI 3" -> [w261]
    tunnel: "HP 1" -> [w260]
    tunnel: "HP 2" -> [w259]
    tunnel: "GPIB HP" -> [w258]
    tunnel: "GPIB HP 2" -> [w257]
    tunnel: "GPIB L 1" -> [w256]
    tunnel: "GPIB L 2" -> [w255]
    tunnel: "GPIB L 3" -> [w254]
    tunnel: "Nr. of Accumulations" -> [w253]
    stop <- w273 continue-if-true
    n109 = stacked-sequence {
      seq-local: [w285 _] -> [_ w354]
      seq-local: [w284 _] -> [_ w355]
      tunnel: w266 -> [w291 _]
      tunnel: w282 -> [w290 _]
      tunnel: w281 -> [w289 _]
      tunnel: w280 -> [w288 _]
      tunnel: w279 -> [w287 _]
      tunnel: w278 -> [w286 _]
      tunnel: [_ w354] -> w267
      tunnel: [_ w355] -> w264
      tunnel: [w283 _] -> w265
      frame #0 {
        # "Read B Field"
        n110 = case shown="0, Default" w291 {
          tunnel: w290 -> [w301 w324]
          tunnel: w289 -> [w300 w323]
          tunnel: w288 -> [w299 w322]
          tunnel: w287 -> [w298 w321]
          tunnel: w286 -> [_ w320]
          tunnel: [w294 w319] -> w285
          tunnel: [w293 w317] -> w284
          tunnel: [w292 w318] -> w283
          frame #0 {
            n111 = call <userlib>:"Get 2D Field (Cartesian).vi"("Y-Axis Communications Config"=w301, "Z-Axis Communications Config"=w300, "error in"=w299) -> ("All Instruments Responded?"=w295:bool, "Y-Axis Field (kG)"=w297:dbl, "Z-Axis Field (kG)"=w296:dbl, "error out"=w294:T5)  [unwired: 2 in]
            n112 = case shown="0, Default" w298 {
              tunnel: w297 -> [w302 w310]
              tunnel: w296 -> [w303 w311]
              tunnel: w295 -> [w304 w313]
              tunnel: [w303 w309] -> w293
              tunnel: [w302 w308] -> w292
              frame #0 {
                n113 = case shown="True" w304 {
                  tunnel: w302 -> [_ w306]
                  tunnel: w303 -> [_ w305]
                  frame #0 {
                  }
                  frame #1 {
                    n114 = Bundle("Y-Axis Field (kG)"=w306, "Z-Axis Field (kG)"=w305) -> (→"Cartesian Display (kG)":T6)  [unwired: 1 in]
                  }
                }
              }
              frame #1 {
                w312 = 0.1 ("y")
                n115 = Multiply(x=w310, y=w312) -> (x*y=w308:dbl)
                n116 = Multiply(x=w311, y=w312) -> (x*y=w309:dbl)
                n117 = case shown="True" w313 {
                  tunnel: w308 -> [_ w316]
                  tunnel: w309 -> [_ w315]
                  frame #0 {
                  }
                  frame #1 {
                    n118 = Bundle(w316, w315) -> (→"Cartesian Display (T)":cluster{dbl, dbl})  [unwired: 1 in]
                  }
                }
              }
            }
          }
          frame #1 {
            n119 = stacked-sequence {
              tunnel: w324 -> [w335]
              tunnel: w323 -> [w334]
              tunnel: w322 -> [w333]
              tunnel: w321 -> [w332]
              tunnel: w320 -> [w329]
              tunnel: [w327] -> w319
              tunnel: [w326] -> w317
              tunnel: [w325] -> w318
              frame #0 {
                # "Field"
                n120 = call <userlib>:"Get 2D Field (Polar).vi"("Y-Axis Communications Config"=w335, "Z-Axis Communications Config"=w334, "error in"=w333) -> ("All Instruments Responded?"=w328:bool, "Radial (r) Field (kG)"=w331:dbl, "q (radians)"=w330:dbl, "error out"=w327:T5)  [unwired: 2 in]
                n121 = case shown="1" w332 {
                  tunnel: w331 -> [w337 w349]
                  tunnel: w330 -> [w339 w348]
                  tunnel: w329 -> [w338 w347]
                  tunnel: w328 -> [w340 w346]
                  tunnel: [w337 w344] -> w326
                  tunnel: [w336 w345] -> w325
                  frame #0 {
                    n122 = Multiply(x=w339, y=w338) -> (x*y=w336:dbl)
                    n123 = case shown="True" w340 {
                      tunnel: w337 -> [_ w341]
                      tunnel: w336 -> [_ w342]
                      frame #0 {
                      }
                      frame #1 {
                        n124 = Bundle(w342, "Radial (r) Field (kG)"=w341) -> (→"Polar Display (kG)":cluster{dbl, "Radial (r) Field (kG)":dbl})  [unwired: 1 in]
                      }
                    }
                  }
                  frame #1 {
                    n125 = Multiply(x=w349, y=0.1) -> (x*y=w345:dbl)
                    n126 = Multiply(x=w348, y=w347) -> (x*y=w344:dbl)
                    n127 = case shown="True" w346 {
                      tunnel: w345 -> [_ w351]
                      tunnel: w344 -> [_ w352]
                      frame #0 {
                      }
                      frame #1 {
                        n128 = Bundle(w352, w351) -> (→"Polar Display (T)":cluster{dbl, dbl})  [unwired: 1 in]
                      }
                    }
                  }
                }
              }
            }
          }
        }
      }
      frame #1 {
        # "Change PID"
        n129 = case shown="True" "Change\nPID\n(DetermineSIMPID.vi)" {
          tunnel: w355 -> [_ w360]
          frame #0 {
          }
          frame #1 {
            # "z Field Value"
            n130 = call "CheckFieldRange.vi"("Field Value"=w360) -> ("Field Range"=w357:dbl)  [unwired: 10 in]
            n131 = Equal?(x="FieldRange", y=w357) -> (x = y?=w359:bool)
            n132 = case shown="False" w359 {
              tunnel: w357 -> [w365 w366]
              frame #0 {
                n133 = local write "FieldRange"(w365) -> ()
                n134 = call "DetermineSIMPID.vi"("Field Range"=w365) -> ("D"=w363:string, "P"=w364:string)  [unwired: 7 in, 2 out]
                n135 = call "SIM960ChangeP.vi"("New D Value"=w363, "New P Value"=w364, "Port Num- PID"="1", "GPIB-Adress"="2") -> ()  [unwired: 8 in]
              }
              frame #1 {
                n136 = local write "FieldRange"(w366) -> ()
              }
            }
          }
        }
      }
    }
    n137 = local read "Ramping Control"() -> (w277:u16)
    n138 = local read "Messfile Refnum"() -> (w252:refnum<file>)
    n139 = case shown="1" w277 {
      selector: w277 -> [w368 w399 w538 w542 w557]
      tunnel: w276 -> [_ w401 _ w545 w562]
      tunnel: w275 -> [_ w400 _ w544 w561]
      tunnel: [w367 w371 w537 w543 w560] -> w274
      tunnel: [w368 w399 w538 w542 w557] -> w272
      tunnel: w271 -> [_ _ _ w541 w559]
      tunnel: w270 -> [_ _ _ _ w556]
      tunnel: w269 -> [_ _ _ _ w555]
      tunnel: w268 -> [_ w391 _ _ _]
      tunnel: w267 -> [w367 w387 w537 w539 w554]
      tunnel: w265 -> [_ w384 _ _ _]
      tunnel: w264 -> [_ w383 _ _ _]
      tunnel: w263 -> [_ w382 _ _ _]
      tunnel: w262 -> [_ w381 _ _ _]
      tunnel: w261 -> [_ w380 _ _ _]
      tunnel: w260 -> [_ w379 _ _ _]
      tunnel: w259 -> [_ w378 _ _ _]
      tunnel: w258 -> [_ w377 _ _ _]
      tunnel: w257 -> [_ w376 _ _ _]
      tunnel: w256 -> [_ w375 _ _ _]
      tunnel: w255 -> [_ w374 _ _ _]
      tunnel: w254 -> [_ w373 _ _ _]
      tunnel: w253 -> [_ w370 _ _ _]
      tunnel: w252 -> [_ w369 _ _ _]
      frame #0 {
      }
      frame #1 {
        w394 = T9."HOLDING" ("y")
        n140 = local read "Number of lines"() -> (w388:i32)
        n141 = local read "Starting index"() -> (w390:i32)
        n142 = call <userlib>:"Get Ramping Mode.vi"("Communications Config"=w401, "error in"=w387) -> ("Ramping Mode"=w397:T10, "error out"=w398:T5)  [unwired: 1 out]
        n143 = call <userlib>:"Get Ramping Mode.vi"("Communications Config"=w400, "error in"=w398) -> ("Ramping Mode"=w396:T10, "error out"=w372:T5)  [unwired: 1 out]
        n144 = Less?(x=w390, y=w388) -> (x < y?=w389:bool)
        n145 = Equal?(x=w397, y=w394) -> (x = y?=w393:bool)
        n146 = Equal?(x=w396, y=w394) -> (x = y?=w392:bool)
        n147 = Compound Arithmetic op=AND(w393, w392) -> (w395:bool)
        n148 = case shown="True" w395 {
          tunnel: w391 -> [_ w422]
          tunnel: w389 -> [_ w421]
          tunnel: "Wait between \nVectors (ms)" -> [_ w420]
          tunnel: "Wait between \nVectors" -> [_ w419]
          tunnel: w384 -> [_ w418]
          tunnel: w383 -> [_ w417]
          tunnel: w382 -> [_ w416]
          tunnel: w381 -> [_ w415]
          tunnel: w380 -> [_ w414]
          tunnel: w379 -> [_ w413]
          tunnel: w378 -> [_ w412]
          tunnel: w377 -> [_ w411]
          tunnel: w376 -> [_ w410]
          tunnel: w375 -> [_ w409]
          tunnel: w374 -> [_ w408]
          tunnel: w373 -> [_ w407]
          tunnel: w372 -> [w402 w406]
          tunnel: [w402 w405] -> w371
          tunnel: w370 -> [_ w404]
          tunnel: w369 -> [_ w403]
          frame #0 {
          }
          frame #1 {
            n149 = case shown="1" w422 {
              tunnel: w421 -> [_ w444]
              tunnel: w420 -> [_ w443]
              tunnel: w419 -> [_ w442]
              tunnel: w418 -> [_ w441]
              tunnel: w417 -> [_ w440]
              tunnel: w416 -> [_ w439]
              tunnel: w415 -> [_ w438]
              tunnel: w414 -> [_ w437]
              tunnel: w413 -> [_ w436]
              tunnel: w412 -> [_ w435]
              tunnel: w411 -> [_ w434]
              tunnel: w410 -> [_ w433]
              tunnel: w409 -> [_ w432]
              tunnel: w408 -> [_ w431]
              tunnel: w407 -> [_ w430]
              tunnel: w406 -> [w423 w429]
              tunnel: [w423 w428] -> w405
              tunnel: w404 -> [_ w427]
              tunnel: w403 -> [_ w426]
              frame #0 {
                w425 = u16 2 items=["NEXT VECTOR", "RAMPING", "HOLDING", "PAUSE", "ZERO"] ("Ramping Control")
                n150 = local write "STATUS"("Holding at current vector. Set Ramping Mode to NEXT VECTOR to continue." ("STATUS")) -> ()
                n151 = local write "Ramping Control"(w425) -> ()
              }
              frame #1 {
                # "Go to NEXT VECTOR automatically"
                n152 = case shown="True" w444 {
                  tunnel: w443 -> [_ w465]
                  tunnel: w442 -> [_ w464]
                  tunnel: w441 -> [_ w463]
                  tunnel: w440 -> [_ w462]
                  tunnel: w439 -> [_ w461]
                  tunnel: w438 -> [_ w460]
                  tunnel: w437 -> [_ w459]
                  tunnel: w436 -> [_ w458]
                  tunnel: w435 -> [_ w457]
                  tunnel: w434 -> [_ w456]
                  tunnel: w433 -> [_ w455]
                  tunnel: w432 -> [_ w454]
                  tunnel: w431 -> [_ w453]
                  tunnel: w430 -> [_ w452]
                  tunnel: w429 -> [w445 w451]
                  tunnel: [w445 w450] -> w428
                  tunnel: w427 -> [_ w449]
                  tunnel: w426 -> [_ w448]
                  frame #0 {
                    w447 = u16 2 items=["NEXT VECTOR", "RAMPING", "HOLDING", "PAUSE", "ZERO"] ("Ramping Control")
                    n153 = local write "STATUS"("Holding at current vector. Set Ramping Mode to NEXT VECTOR to continue." ("STATUS")) -> ()
                    n154 = local write "Ramping Control"(w447) -> ()
                  }
                  frame #1 {
                    n155 = stacked-sequence {
                      tunnel: w465 -> [w483 _]
                      tunnel: w464 -> [w482 _]
                      tunnel: w463 -> [w481 _]
                      tunnel: w462 -> [w480 _]
                      tunnel: w461 -> [w479 _]
                      tunnel: w460 -> [w478 _]
                      tunnel: w459 -> [w477 _]
                      tunnel: w458 -> [w476 _]
                      tunnel: w457 -> [w475 _]
                      tunnel: w456 -> [w474 _]
                      tunnel: w455 -> [w473 _]
                      tunnel: w454 -> [w472 _]
                      tunnel: w453 -> [w471 _]
                      tunnel: w452 -> [w470 _]
                      tunnel: w451 -> [w469 _]
                      tunnel: [w468 _] -> w450
                      tunnel: w449 -> [w467 _]
                      tunnel: w448 -> [w466 _]
                      frame #0 {
                        n156 = case shown="False" w482 {
                          tunnel: w483 -> [_ w501]
                          tunnel: w481 -> [_ w500]
                          tunnel: w480 -> [_ w499]
                          tunnel: w479 -> [_ w498]
                          tunnel: w478 -> [_ w497]
                          tunnel: w477 -> [_ w496]
                          tunnel: w476 -> [_ w495]
                          tunnel: w475 -> [_ w494]
                          tunnel: w474 -> [_ w493]
                          tunnel: w473 -> [_ w492]
                          tunnel: w472 -> [_ w491]
                          tunnel: w471 -> [_ w490]
                          tunnel: w470 -> [_ w489]
                          tunnel: w469 -> [w484 w488]
                          tunnel: [w484 w487] -> w468
                          tunnel: w467 -> [_ w486]
                          tunnel: w466 -> [_ w485]
                          frame #0 {
                          }
                          frame #1 {
                            n157 = stacked-sequence {
                              tunnel: w501 -> [w502 _]
                              tunnel: w500 -> [_ w534]
                              tunnel: w499 -> [_ w533]
                              tunnel: [_ w503] -> _
                              tunnel: w498 -> [_ w532]
                              tunnel: w497 -> [_ w531]
                              tunnel: w496 -> [_ w530]
                              tunnel: w495 -> [_ w529]
                              tunnel: w494 -> [_ w528]
                              tunnel: w493 -> [_ w527]
                              tunnel: w492 -> [_ w526]
                              tunnel: w491 -> [_ w525]
                              tunnel: w490 -> [_ w524]
                              tunnel: w489 -> [_ w523]
                              tunnel: w488 -> [_ w522]
                              tunnel: [_ w507] -> w487
                              tunnel: w486 -> [_ w506]
                              tunnel: w485 -> [_ w503]
                              frame #0 {
                                n158 = Wait (ms)(milliseconds to wait=w502) -> ()  [unwired: 1 out]
                              }
                              frame #1 {
                                n159 = call "ReadallDevicesv1.vi"("GPIB HP 2"=w526, "LI 3"=w530, "LI 2"=w531, "LI 1"=w532, "Nr. of Accumulations"=w506, "HP 2"=w528, "GPIB HP"=w527, "Y-Axis Field (kG)"=w534, "HP 1"=w529, "Radial (r) Field (kG) 2"=w533, "error in"=w522, "GPIB L 3"=w523, "GPIB L 2"=w524, "GPIB L 1"=w525) -> ("appended array"=w504:dbl[], "error out"=w508:errorcluster)
                                "appended array" <- w504
                                n160 = Array To Spreadsheet String(array=w504, 3:"%f" ("format string")) -> (spreadsheet string=w509:string)  [unwired: 1 in]
                                n161 = local read "measured data"() -> (w521:dbl[][])
                                n162 = Insert Into Array(array=w521, new element=w504) -> (w505:dbl[][])  [unwired: 2 in]
                                n163 = Index Array(array=w505, index (col)="X Axis") -> (element=w520:dbl[])  [unwired: 1 in]
                                n164 = Index Array(array=w505, index (col)="Y Axis") -> (element=w519:dbl[])  [unwired: 1 in]
                                n165 = Set File Position(refnum=w503, from (0:start)=1, error in=w508) -> (refnum out=w514:refnum<file>, error out=w513:errorcluster)  [unwired: 1 in]
                                n166 = Bundle("measured data"=w520, "measured data"=w519) -> (w518:T2)  [unwired: 1 in]
                                n167 = local write "measured data"(w505) -> ()
                                n168 = Write to Text File(file (use dialog)=w514, text=w509, error in=w513) -> (refnum out=w511:refnum<file>, error out=w512:errorcluster)  [unwired: 1 in, 1 out]
                                n169 = local write "XY Graph"(w518) -> ()
                                n170 = Flush File(refnum=w511, error in=w512) -> (error out=w507:errorcluster)  [unwired: 1 out]
                              }
                            }
                          }
                        }
                      }
                      frame #1 {
                        w536 = u16 0 items=["NEXT VECTOR", "RAMPING", "HOLDING", "PAUSE", "ZERO"] ("Ramping Control")
                        n171 = local write "Ramping Control"(w536) -> ()
                        n172 = local write "STATUS"("Go to NEXT VECTOR" ("STATUS")) -> ()
                      }
                    }
                  }
                }
              }
            }
          }
        }
      }
      frame #2 {
      }
      frame #3 {
        n173 = Not Equal?(x=w542, y=w541) -> (x != y?=w540:bool)
        n174 = case shown="False" w540 {
          tunnel: w545 -> [_ w553]
          tunnel: w544 -> [_ w552]
          tunnel: [w546 w550] -> w543
          tunnel: w539 -> [w546 w547]
          frame #0 {
          }
          frame #1 {
            w548 = u16 1 items=["RAMP", "PAUSE", "MANUAL UP", "MANUAL DOWN", "ZERO"] ("Ramping Mode")
            n175 = call <userlib>:"Set Ramping Mode.vi"("error in"=w547, "Ramping Mode"=w548, "Communications Config"=w553) -> ("error out"=w551:T5)
            n176 = call <userlib>:"Set Ramping Mode.vi"("error in"=w551, "Ramping Mode"=w548, "Communications Config"=w552) -> ("error out"=w550:T5)
            n177 = local write "STATUS"("All Programmers are PAUSED. Set Ramping Mode to NEXT VECTOR to continue." ("STATUS")) -> ()
          }
        }
      }
      frame #4 {
        n178 = Not Equal?(x=w557, y=w559) -> (x != y?=w558:bool)
        n179 = case shown="False" w558 {
          tunnel: w562 -> [_ w571]
          tunnel: w561 -> [_ w570]
          tunnel: [w563 w566] -> w560
          tunnel: w556 -> [_ w569]
          tunnel: w555 -> [_ w568]
          tunnel: w554 -> [w563 w564]
          frame #0 {
          }
          frame #1 {
            w565 = u16 4 items=["RAMP", "PAUSE", "MANUAL UP", "MANUAL DOWN", "ZERO"] ("Ramping Mode")
            n180 = local write "STATUS"("Zeroing vector." ("STATUS")) -> ()
            n181 = call <userlib>:"Set Ramping Mode.vi"("error in"=w564, "Ramping Mode"=w565, "Communications Config"=w571) -> ("error out"=w574:T5)
            n182 = call <userlib>:"Set Ramping Mode.vi"("error in"=w574, "Ramping Mode"=w565, "Communications Config"=w570) -> ("error out"=w567:T5)
            n183 = call <userlib>:"Set Current Ramp Rate.vi"("Communications Config"=w571, "Ramp Rate (A/sec)"=w569, "error in"=w567) -> ("error out"=w572:T5)  [unwired: 2 in]
            n184 = call <userlib>:"Set Current Ramp Rate.vi"("Communications Config"=w570, "Ramp Rate (A/sec)"=w568, "error in"=w572) -> ("error out"=w566:T5)  [unwired: 2 in]
          }
        }
      }
    }
    n185 = local read "Continue Execution?"() -> (w273:bool)
  }
  n186 = case shown="0, Default" w40 {
    tunnel: w36 -> [w577 _ _]
    tunnel: w34 -> [w576 w580 w581]
    tunnel: [w575 w579 w581] -> w41
    tunnel: w35 -> [_ w578 _]
    frame #0 {
      n187 = call <userlib>:"430_TCP_Close.vi"("error in (no error)"=w576, "connection ID"=w577) -> ("error out"=w575:errorcluster)  [unwired: 1 out]
    }
    frame #1 {
      n188 = call <userlib>:"430_RS232_Close.vi"("error in (no error)"=w580, "VISA resource name"=w578) -> ("error out"=w579:errorcluster)  [unwired: 1 in]
    }
    frame #2 {
    }
  }
  n189 = case shown="0, Default" w39 {
    tunnel: w38 -> [w584 _ _]
    tunnel: w41 -> [w583 w587 w588]
    tunnel: [w582 w586 w588] -> w31
    tunnel: w37 -> [_ w585 _]
    frame #0 {
      n190 = call <userlib>:"430_TCP_Close.vi"("error in (no error)"=w583, "connection ID"=w584) -> ("error out"=w582:errorcluster)  [unwired: 1 out]
    }
    frame #1 {
      n191 = call <userlib>:"430_RS232_Close.vi"("error in (no error)"=w587, "VISA resource name"=w585) -> ("error out"=w586:errorcluster)  [unwired: 1 in]
    }
    frame #2 {
    }
  }
  "error out" <- w31
  n192 = local read "Magnetic Field Units"() -> (w58:u16)
  n193 = local read "Coordinate System"() -> (w59:u16)
  n194 = while {
    tunnel: "Starting index" -> [w596]
    tunnel: w33 -> [w602]
    tunnel: w32 -> [w603]
    tunnel: w58 -> [w604]
    tunnel: w59 -> [w605]
    tunnel: w56 -> [w608]
    tunnel: "Max Ramp Rate - Y Axis (A/s)" -> [w592]
    tunnel: "Max Ramp Rate - Z Axis (A/s)" -> [w591]
    tunnel: "Magnitude Limit (kG)" -> [w593]
    tunnel: "User defined Ramp Rate (T/min)" -> [w590]
    tunnel: "User defined Ramp Rate (T/min)" -> [w589]
    i -> [w595]
    stop <- w597 continue-if-true
    n195 = local read "Field Values"() -> (w599:string[][])
    n196 = Add(x=w596, y=w595) -> (x+y=w594:i32)
    n197 = while "Wait for NEXT VECTOR setting by operator." {
      tunnel: [w612] -> w607
      tunnel: w608 -> [w612]
      stop <- w613 continue-if-true
      w611 = u16 0 items=["NEXT VECTOR", "RAMPING", "HOLDING", "PAUSE", "ZERO"] ("Ramping Control")
      n198 = local read "Ramping Control"() -> (w614:u16)
      n199 = Not Equal?(x=w611, y=w614) -> (x != y?=w613:bool)
    }
    n200 = stacked-sequence {
      tunnel: w594 -> [w616 _ w622 _]
      frame #0 {
        (unwired) -2
        n201 = Subtract(x=w616, y=2) -> (x-y=w619:i32)
        n202 = Bundle(w619, -2) -> (w617:cluster{i32, i32})  [unwired: 1 in]
        n203 = property on="Field Values" class="Tbl (strict)"("Active Cell:Active Cell"=w617) -> ()  [unwired: 2 in, 2 out]
      }
      frame #1 {
        n204 = local read "Normal color"() -> (w620:u32)
        n205 = property on="Field Values" class="Tbl (strict)"("Active Cell:Cell Background Color"=w620) -> ()  [unwired: 2 in, 2 out]
      }
      frame #2 {
        n206 = Decrement(x=w622) -> (x-1=w621:i32)
        n207 = Bundle(w621, -2) -> (w624:cluster{i32, i32})  [unwired: 1 in]
        n208 = property on="Field Values" class="Tbl (strict)"("Active Cell:Active Cell"=w624) -> ()  [unwired: 2 in, 2 out]
      }
      frame #3 {
        n209 = property on="Field Values" class="Tbl (strict)"("Active Cell:Cell Background Color"="Highlight color") -> ()  [unwired: 2 in, 2 out]
      }
    }
    n210 = Index Array(array=w599, index (row)=w594) -> (element=w606:string[])  [unwired: 1 in]
    n211 = local write "Starting index"(w594) -> ()
    n212 = Add(x=1, y=w594) -> (x+y=w609:i32)
    n213 = Number To Decimal String(number=w609) -> (decimal integer string=w598:string)  [unwired: 1 in]
    n214 = stacked-sequence {
      tunnel: [_ w650] -> w600
      tunnel: [_ w649] -> w601
      tunnel: w607 -> [_ w645]
      tunnel: w606 -> [_ w644]
      tunnel: w605 -> [_ w643]
      tunnel: w604 -> [_ w642]
      tunnel: w603 -> [_ w641]
      tunnel: w602 -> [_ w640]
      tunnel: w598 -> [_ w639]
      tunnel: w593 -> [_ w637]
      tunnel: w592 -> [_ w636]
      tunnel: w591 -> [_ w631]
      tunnel: w590 -> [_ w635]
      tunnel: w589 -> [_ w634]
      frame #0 {
        w629 = u16 1 items=["NEXT VECTOR", "RAMPING", "HOLDING", "PAUSE", "ZERO"] ("Ramping Control")
        n215 = local write "Ramping Control"(w629) -> ()
      }
      frame #1 {
        n216 = call <userlib>:"Set 2D Next Vector_entwurf.vi"("Coordinate System"=w643, "Magnetic Field Units"=w642, 3:"User defined Ramp Rate (T/min)"=w634, "Magnitude Limit (kG)"=w637, "Y-Axis Communications Config"=w641, "Input Vector"=w644, "Z-Axis Communications Config"=w640, 10:"User defined Ramp Rate (T/min)"=w635, "Max Ramp Rate - Y Axis (A/s)"=w636, "error in"=w645, "Max Ramp Rate - Z Axis (A/s)"=w631) -> ("Y-Axis Ramp Rate (T/min)"=→"Current Ramp Rate Y (T/min)":dbl, "Within Limits?"=w650:bool, "Ramp Rate along Vector (T/min)"=→"Ramp Rate along Vector (T/min)":dbl, "Z-Axis Ramp Rate (T/min)"=→"Current Ramp Rate Z (T/min)":dbl, "All Instruments Responded?"=w649:bool, "error out"=w638:T5)  [unwired: 3 in]
        n217 = Concatenate Strings("Ramping to field vector " ("STATUS"), w639, "..." ("STATUS")) -> (w646:string)
        n218 = local write "error in"(w638) -> ()
        n219 = local write "STATUS"(w646) -> ()
      }
    }
    n220 = case shown="True" w600 {
      tunnel: w601 -> [_ w627]
      frame #0 {
        n221 = local write "STATUS"("Vector magnitude limt or maximum coil current exceeded. Vector ignored. VI halted." ("STATUS")) -> ()
      }
      frame #1 {
        n222 = case shown="True" w627 {
          frame #0 {
            n223 = local write "STATUS"("Not all programmers responded. VI halted." ("STATUS")) -> ()
          }
          frame #1 {
          }
        }
      }
    }
    n224 = Compound Arithmetic op=AND(w601, w600) -> (w597:bool)
    n225 = local write "Continue Execution?"(w597) -> ()
  }
